vi "get-color-submatrix.vi"(9 "Value":u8, 10 "Real Matrix in":T2, 11 "image data":T1) -> (3 "Real Matrix out":T2)   [LabVIEW 2016]
uses:
  <vilib>/Analysis/Matrix/Datatypes/RealMatrix.ctl
  <vilib>/picture/picture.llb/imagedata.ctl
  <vilib>/Analysis/Matrix/NI_Matrix.lvlib
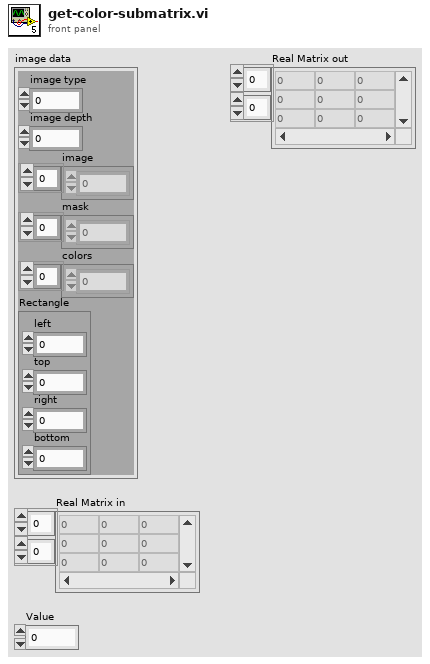
[diagram p1: front panel]
types:
  T1 = typedef "imagedata.ctl" = cluster{"image type":i32, "image depth":i32, "image":u8[], "mask":u8[], "colors":u32[], "Rectangle":cluster{"left":i16, "top":i16, "right":i16, "bottom":i16}}
  T2 = typedef "NI_Matrix.lvlib/RealMatrix.ctl" = dbl[][]
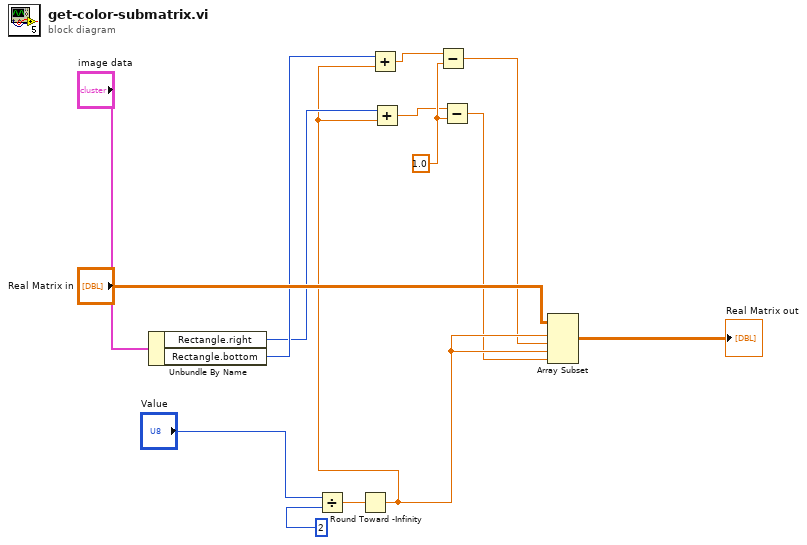
[diagram p0: block diagram]
diagram:
  w8 = 1.0 ("y")
  n1 = Unbundle By Name("image data") -> ("Rectangle.right"=w4:i16, "Rectangle.bottom"=w5:i16)
  n2 = Divide(x="Value", y=u8 2) -> (x/y=w9:dbl)
  n3 = Round Toward -Infinity(1:w9) -> (0:w3:dbl)
  n4 = Add(x=w5, y=w3) -> (x+y=w7:dbl)
  n5 = Add(x=w4, y=w3) -> (x+y=w6:dbl)
  n6 = Subtract(x=w7, y=w8) -> (x-y=w2:dbl)
  n7 = Subtract(x=w6, y=w8) -> (x-y=w1:dbl)
  n8 = Array Subset(array="Real Matrix in", index (row)=w3, length (row)=w2, index (col)=w3, length (col)=w1) -> (→"Real Matrix out":T2)
